vi "Read Anything.vi"(7 "Type of Anything":variant, 8 "Error In":errorcluster, 9 "Section Name (Name of \"Type of Anything\")":string, 11 "Path (dialog)":path) -> (0 "Error Out":errorcluster, 1 "Found?":bool, 3 "Anything":variant)   [LabVIEW 2009]
doc: "This VI is designed to read data from a file written by <B>Write Anything.vi</B>. If the data type definition has changed since it was written to file, this VI will still read and fill out any elements of the cluster that have the same name. Any elements for which it cannot find a name match in the file will be supplied with their datatype's default value.\n\nFreeware from Moore Good Ideas, www.mooregoodideas.com. Do not remove this line."
uses:
  <vilib>/Utility/VariantDataType/VariantType.lvlib
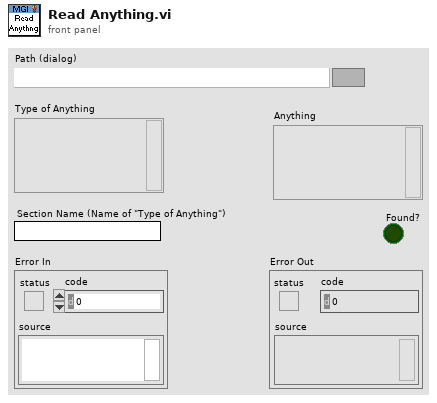
[diagram p1: front panel]
types:
  T1 = typedef "VariantType.lvlib/Type.ctl" = enum8{"Invalid Type", "Void", "I8", "I16", "I32", "I64", "U8", "U16", "U32", "U64", "Single Float", "Double Float", "Extended Float", "Single Complex", "Double Complex", "Extended Complex", "Enum U8", "Enum U16", "Enum U32", "Enum U64", "Single Float With Unit", "Double Float With Unit", "Extended Float With Unit", "Single Complex with Unit", "Double Complex with Unit", "Extended Complex with Unit", "Boolean", "String", "Path", "Picture", "Tag", "Array", "Cluster", "Variant", "LV Variant", "Waveform", "Timestamp", "Digital Waveform", "Digital Data", "ExpressData", "Refnum", "External Data", "VI", "Poly VI", "LabVIEW Class Instance", "Fixed Point"}
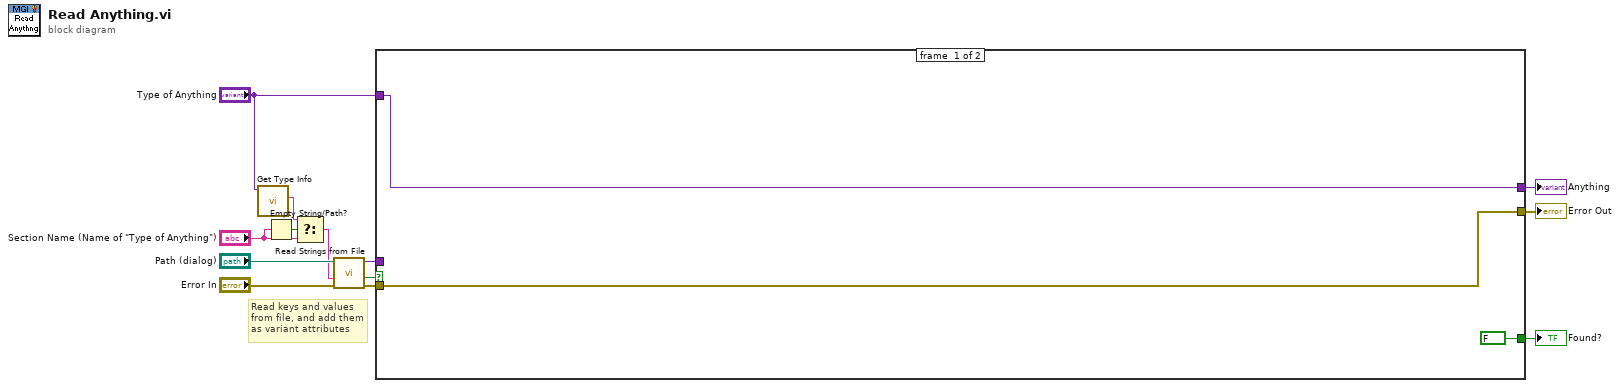
[diagram p0: block diagram]
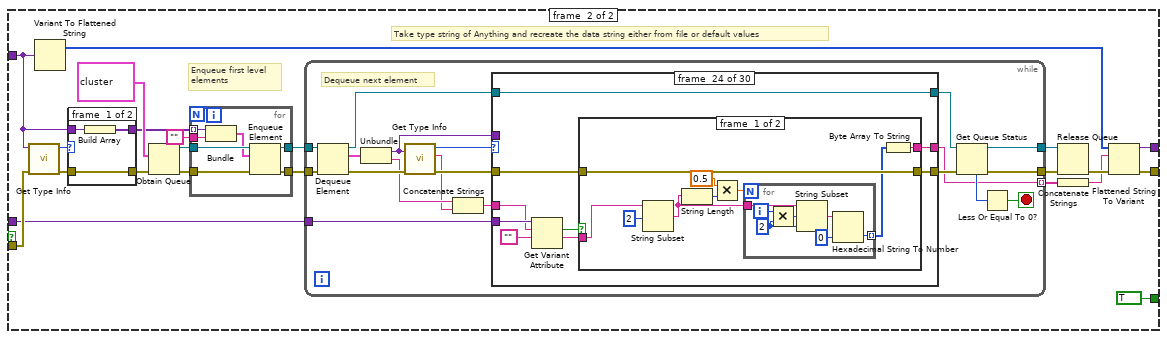
[diagram p2: hidden frame]
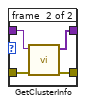
[diagram p3: hidden frame]
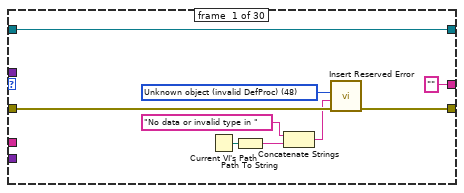
[diagram p4: hidden frame]
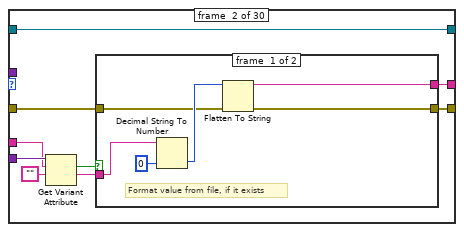
[diagram p5: hidden frame]
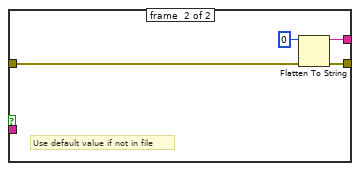
[diagram p6: hidden frame]
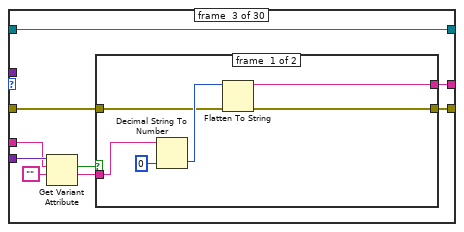
[diagram p7: hidden frame]
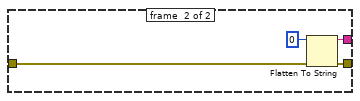
[diagram p8: hidden frame]
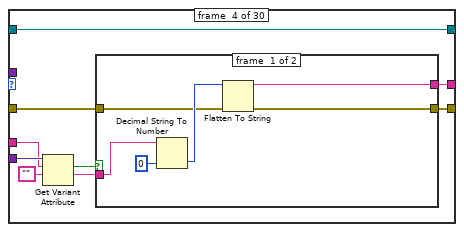
[diagram p9: hidden frame]
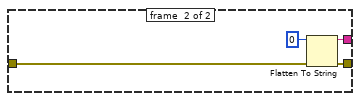
[diagram p10: hidden frame]
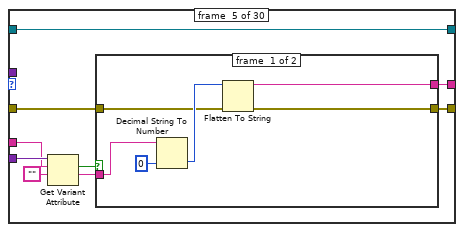
[diagram p11: hidden frame]
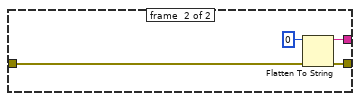
[diagram p12: hidden frame]
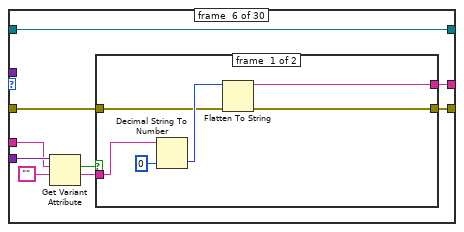
[diagram p13: hidden frame]
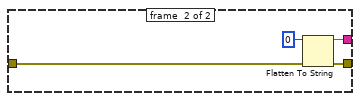
[diagram p14: hidden frame]
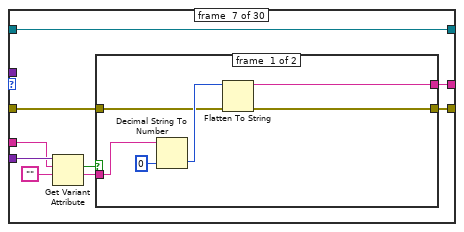
[diagram p15: hidden frame]
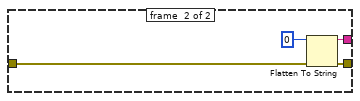
[diagram p16: hidden frame]
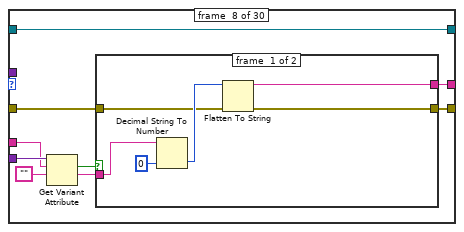
[diagram p17: hidden frame]
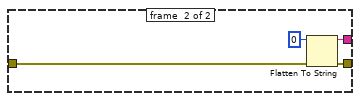
[diagram p18: hidden frame]
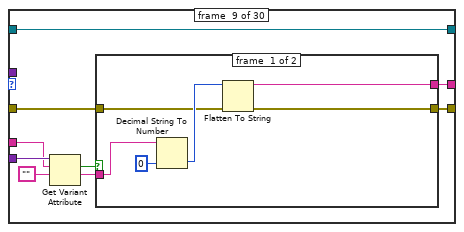
[diagram p19: hidden frame]
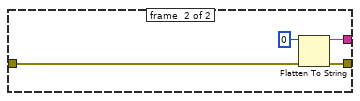
[diagram p20: hidden frame]
diagram:
  # "Read keys and values from file, and add them as variant attributes"
  n1 = call "Get Type Info.vi"("Variant"="Type of Anything") -> ("Name"=w2:string)  [unwired: 8 in, 2 out]
  n2 = Empty String/Path?(string/path="Section Name (Name of \"Type of Anything\")") -> (empty?=w5:bool)
  n3 = Select(t=w2, s=w5, f="Section Name (Name of \"Type of Anything\")") -> (s? t:f=w3:string)
  n4 = call "Read Strings from File.vi"("Error In"="Error In", "Section Name"=w3, "Path"="Path (dialog)") -> ("Error Out"=w11:errorcluster, "Found?"=w8:bool, "Variant Database"=w7:variant)  [unwired: 6 in]
  n5 = case shown="True" w8 {
    tunnel: [w15 w37] -> w13
    tunnel: [w16 w36] -> w12
    tunnel: "Type of Anything" -> [w16 w18]
    tunnel: w11 -> [w15 w24]
    tunnel: [FALSE TRUE] -> w9
    tunnel: w7 -> [_ w22]
    frame #0 {
    }
    frame #1 {
      # "Enqueue first level\nelements"
      # "Take type string of Anything and recreate the data string either from file or default values"
      n6 = call "Get Type Info.vi"("Error In"=w24, "Variant"=w18) -> ("Error Out"=w19:errorcluster, "Type Enum"=w21:T1)  [unwired: 7 in, 1 out]
      n7 = Variant To Flattened String(Variant=w18) -> (1:w38:i16[])  [unwired: 1 out]
      n8 = case shown="\"Cluster\"" w21 {
        tunnel: [w41 w44] -> w20
        tunnel: w19 -> [w41 w45]
        tunnel: w18 -> [w40 w43]
        tunnel: [w39 w42] -> w17
        frame #0 {
          n9 = Build Array(w40) -> (w39:variant[])
        }
        frame #1 {
          n10 = call <vilib>:"GetClusterInfo.vi"("error in (no error)"=w45, "Variant"=w43) -> ("error out"=w44:errorcluster, "Cluster Elements"=w42:variant[])  [unwired: 8 in]
        }
      }
      n11 = Obtain Queue(element data type=cluster{"Variant":variant, "Name":string} {"Variant"=variant, "Name"=""}, error in (no error)=w20) -> (queue out=w34:refnum<queue>, error out=w26:errorcluster)  [unwired: 3 in, 1 out]
      n12 = for {
        tunnel: w34 -> [w52]
        tunnel: [w51] -> w33
        tunnel: [w50] -> w32
        tunnel: w17 -> [w49] mode=indexing
        tunnel: "" -> [w47]
        tunnel: w26 -> [w46]
        n13 = Bundle("ArrayElt"=w49, w47) -> (w48:cluster{"ArrayElt":variant, string})  [unwired: 1 in]
        n14 = Enqueue Element(queue=w52, element=w48, error in (no error)=w46) -> (queue out=w50:refnum<queue>, error out=w51:errorcluster)  [unwired: 1 in, 1 out]
      }
      n15 = while {
        tunnel: w33 -> [w69]
        tunnel: [w64] -> w31
        tunnel: w22 -> [w56]
        tunnel: [w53] -> w35 mode=indexing
        tunnel: w32 -> [w66]
        tunnel: [w60] -> w29
        stop <- w61 stop-if-true
        # "Dequeue next element"
        n16 = Dequeue Element(queue=w66, error in (no error)=w69) -> (queue out=w67:refnum<queue>, element=w59:cluster{"Variant":variant, "Name":string}, error out=w68:errorcluster)  [unwired: 1 in, 1 out]
        n17 = Unbundle(w59) -> ("Variant"=w55:variant, "Name"=w57:string)
        n18 = call "Get Type Info.vi"("Error In"=w68, "Variant"=w55) -> ("Error Out"=w70:errorcluster, "Name"=w54:string, "Type Enum"=w71:T1)  [unwired: 7 in]
        n19 = Concatenate Strings(w57, w54) -> (w58:string)
        n20 = case shown="\"Invalid Type\", \"Void\"" w71 {
          tunnel: [w74 w89 w108 w127 w146 w165 w184 w203 w222 w241 w260 w279 w298 w317 w336 w356 w382 w408 w434 w459 w478 w495 w510 w532 w561 w590 w619 w648 w676 w688] -> w65
          tunnel: w70 -> [w75 w88 w107 w126 w145 w164 w183 w202 w221 w240 w259 w278 w297 w316 w335 w355 w381 w407 w433 w458 w477 w494 w516 w531 w560 w589 w618 w647 w677 w687]
          tunnel: w58 -> [_ w83 w102 w121 w140 w159 w177 w197 w216 w235 w253 w273 w291 w311 w331 w348 w374 w401 w427 w453 w472 w488 w506 w526 w555 w583 w611 w641 w671 w680]
          tunnel: ["" ("data string") w87 w106 w125 w144 w163 w182 w201 w220 w239 w258 w277 w296 w315 w334 w354 w380 w406 w432 w457 w476 w493 "" w530 w559 w588 w617 w646 w674 w686] -> w53
          tunnel: w55 -> [_ _ _ _ _ _ _ _ _ _ _ _ _ _ _ w353 w379 w405 w431 _ _ _ w515 _ _ _ _ _ w675 _]
          tunnel: w67 -> [w76 w86 w105 w124 w143 w162 w181 w200 w219 w238 w257 w276 w295 w314 w333 w352 w378 w404 w430 w456 w475 w492 w511 w529 w558 w587 w616 w645 w679 w685]
          tunnel: [w76 w86 w105 w124 w143 w162 w181 w200 w219 w238 w257 w276 w295 w314 w333 w352 w378 w404 w430 w456 w475 w492 w509 w529 w558 w587 w616 w645 w678 w685] -> w63
          tunnel: w56 -> [_ w84 w103 w122 w141 w160 w178 w198 w217 w237 w254 w274 w292 w312 w332 w350 w375 w402 w428 w454 w473 w489 _ w527 w556 w585 w614 w642 w672 w683]
          frame #0 {
            w72 = u16 48 items=["No error", "Argument error", "Memory is full", "Out of zone", "End of file", "File already open", "Generic file I/O error", "File not found", "File permission error", "Disk is full", "Duplicate path", "Too many files open", "System feature not enabled", "Resource file not found", "Cannot add resource", "Resource not found", "Image not found", "Image memory error", "Pen does not exist", "Config type invalid", "Config token not found", "Config parse error", "Config memory error", "Bad external code format", "Bad external code offset", "External code not present", "Null window", "Destroy window error", "Null menu", "Print aborted", "Bad print record", "Print driver error", "Windows error during printing", "Memory error during printing", "Print dialog error", "Generic print error", "Invalid device refnum", "Device not found", "Device parameter error", "Device unit error", "Cannot open device", "Device call aborted", "Generic error", "Cancelled by user", "Object ID too low", "Object ID too high", "Object not in heap", "Unknown heap", "Unknown object (invalid DefProc)", "Unknown object (DefProc not in table)", "Message out of range", "Invalid (null) method", "Unknown message", "Manager call not supported", "Bad address", "Network operation in progress", "Network operation timed out", "Connection is busy", "Network attribute not supported", "Network error", "Address in use", "System out of memory", "Connection aborted", "Connection refused", "Not connected", "Already connected", "Connection closed", "Initialization error (interapplication manager)", "Bad occurrence", "Wait on unbound occurrence handler", "Occurrence queue overflow", "Datalog type conflict", "Unused", "Unrecognized type (interapplication manager)", "Memory corrupt", "Failed to make temporary DLL", "Old CIN version", "Drag socket not found", "Failed to load drop-object", "Failed to register OLE object", "Failed to release OLE object", "Format specifier type mismatch", "Unknown format specifier", "Too few format specifiers", "Too many format specifiers", "Scan failed", "Newer CIN version", "OLE Convert", "Runtime menu error", "Password tampered", "Unknown error code"] ("Reserved Error Code")
            n21 = Current VI's Path() -> (path=w78:path)
            n22 = Path To String(path=w78) -> (string=w77:string)
            n23 = Concatenate Strings("No data or invalid type in " ("string"), w77) -> (w73:string)
            n24 = call "Insert Reserved Error.vi"("error in (no error)"=w75, "non-standard source (\"\")"=w73, "Reserved Error Code"=w72) -> ("error out"=w74:errorcluster)  [unwired: 4 in]
          }
          frame #1 {
            n25 = Get Variant Attribute(Variant=w84, name=w83, default value (empty Variant)="") -> (found=w81:bool, value=w82:string)  [unwired: 1 in, 2 out]
            n26 = case shown="True" w81 {
              tunnel: w82 -> [w90 _]
              tunnel: [w93 w96] -> w89
              tunnel: w88 -> [w92 w97]
              tunnel: [w94 w99] -> w87
              frame #0 {
                # "Format value from file, if it exists"
                n27 = Decimal String To Number(string=w90, default (0L)=i8 0 ("default (0 I32)")) -> (number=w95:i8)  [unwired: 1 in, 1 out]
                n28 = Flatten To String(anything=w95, error in (no error)=w92) -> (data string=w94:string, error out=w93:errorcluster)  [unwired: 2 in, 1 out]
              }
              frame #1 {
                # "Use default value if not in file"
                n29 = Flatten To String(anything=i8 0, error in (no error)=w97) -> (data string=w99:string, error out=w96:errorcluster)  [unwired: 2 in, 1 out]
              }
            }
          }
          frame #2 {
            n30 = Get Variant Attribute(Variant=w103, name=w102, default value (empty Variant)="") -> (found=w100:bool, value=w101:string)  [unwired: 1 in, 2 out]
            n31 = case shown="True" w100 {
              tunnel: w101 -> [w109 _]
              tunnel: [w112 w115] -> w108
              tunnel: w107 -> [w111 w116]
              tunnel: [w113 w118] -> w106
              frame #0 {
                n32 = Decimal String To Number(string=w109, default (0L)=i16 0 ("default (0 I32)")) -> (number=w114:i16)  [unwired: 1 in, 1 out]
                n33 = Flatten To String(anything=w114, error in (no error)=w111) -> (data string=w113:string, error out=w112:errorcluster)  [unwired: 2 in, 1 out]
              }
              frame #1 {
                n34 = Flatten To String(anything=i16 0, error in (no error)=w116) -> (data string=w118:string, error out=w115:errorcluster)  [unwired: 2 in, 1 out]
              }
            }
          }
          frame #3 {
            n35 = Get Variant Attribute(Variant=w122, name=w121, default value (empty Variant)="") -> (found=w119:bool, value=w120:string)  [unwired: 1 in, 2 out]
            n36 = case shown="True" w119 {
              tunnel: w120 -> [w128 _]
              tunnel: [w131 w134] -> w127
              tunnel: w126 -> [w130 w135]
              tunnel: [w132 w137] -> w125
              frame #0 {
                n37 = Decimal String To Number(string=w128, default (0L)=0 ("default (0 I32)")) -> (number=w133:i32)  [unwired: 1 in, 1 out]
                n38 = Flatten To String(anything=w133, error in (no error)=w130) -> (data string=w132:string, error out=w131:errorcluster)  [unwired: 2 in, 1 out]
              }
              frame #1 {
                n39 = Flatten To String(anything=0, error in (no error)=w135) -> (data string=w137:string, error out=w134:errorcluster)  [unwired: 2 in, 1 out]
              }
            }
          }
          frame #4 {
            n40 = Get Variant Attribute(Variant=w141, name=w140, default value (empty Variant)="") -> (found=w138:bool, value=w139:string)  [unwired: 1 in, 2 out]
            n41 = case shown="True" w138 {
              tunnel: w139 -> [w147 _]
              tunnel: [w150 w153] -> w146
              tunnel: w145 -> [w149 w154]
              tunnel: [w151 w156] -> w144
              frame #0 {
                n42 = Decimal String To Number(string=w147, default (0L)=i64 0 ("default (0 I32)")) -> (number=w152:i64)  [unwired: 1 in, 1 out]
                n43 = Flatten To String(anything=w152, error in (no error)=w149) -> (data string=w151:string, error out=w150:errorcluster)  [unwired: 2 in, 1 out]
              }
              frame #1 {
                n44 = Flatten To String(anything=i64 0, error in (no error)=w154) -> (data string=w156:string, error out=w153:errorcluster)  [unwired: 2 in, 1 out]
              }
            }
          }
          frame #5 {
            n45 = Get Variant Attribute(Variant=w160, name=w159, default value (empty Variant)="") -> (found=w157:bool, value=w158:string)  [unwired: 1 in, 2 out]
            n46 = case shown="True" w157 {
              tunnel: w158 -> [w166 _]
              tunnel: [w169 w172] -> w165
              tunnel: w164 -> [w168 w173]
              tunnel: [w170 w175] -> w163
              frame #0 {
                n47 = Decimal String To Number(string=w166, default (0L)=u8 0 ("default (0 I32)")) -> (number=w171:u8)  [unwired: 1 in, 1 out]
                n48 = Flatten To String(anything=w171, error in (no error)=w168) -> (data string=w170:string, error out=w169:errorcluster)  [unwired: 2 in, 1 out]
              }
              frame #1 {
                n49 = Flatten To String(anything=u8 0, error in (no error)=w173) -> (data string=w175:string, error out=w172:errorcluster)  [unwired: 2 in, 1 out]
              }
            }
          }
          frame #6 {
            n50 = Get Variant Attribute(Variant=w178, name=w177, default value (empty Variant)="") -> (found=w176:bool, value=w179:string)  [unwired: 1 in, 2 out]
            n51 = case shown="True" w176 {
              tunnel: w179 -> [w185 _]
              tunnel: [w188 w191] -> w184
              tunnel: w183 -> [w187 w192]
              tunnel: [w189 w194] -> w182
              frame #0 {
                n52 = Decimal String To Number(string=w185, default (0L)=u16 0 ("default (0 I32)")) -> (number=w190:u16)  [unwired: 1 in, 1 out]
                n53 = Flatten To String(anything=w190, error in (no error)=w187) -> (data string=w189:string, error out=w188:errorcluster)  [unwired: 2 in, 1 out]
              }
              frame #1 {
                n54 = Flatten To String(anything=u16 0, error in (no error)=w192) -> (data string=w194:string, error out=w191:errorcluster)  [unwired: 2 in, 1 out]
              }
            }
          }
          frame #7 {
            n55 = Get Variant Attribute(Variant=w198, name=w197, default value (empty Variant)="") -> (found=w195:bool, value=w196:string)  [unwired: 1 in, 2 out]
            n56 = case shown="True" w195 {
              tunnel: w196 -> [w204 _]
              tunnel: [w207 w210] -> w203
              tunnel: w202 -> [w206 w211]
              tunnel: [w208 w213] -> w201
              frame #0 {
                n57 = Decimal String To Number(string=w204, default (0L)=u32 0 ("default (0 I32)")) -> (number=w209:u32)  [unwired: 1 in, 1 out]
                n58 = Flatten To String(anything=w209, error in (no error)=w206) -> (data string=w208:string, error out=w207:errorcluster)  [unwired: 2 in, 1 out]
              }
              frame #1 {
                n59 = Flatten To String(anything=u32 0, error in (no error)=w211) -> (data string=w213:string, error out=w210:errorcluster)  [unwired: 2 in, 1 out]
              }
            }
          }
          frame #8 {
            n60 = Get Variant Attribute(Variant=w217, name=w216, default value (empty Variant)="") -> (found=w214:bool, value=w215:string)  [unwired: 1 in, 2 out]
            n61 = case shown="True" w214 {
              tunnel: w215 -> [w223 _]
              tunnel: [w226 w229] -> w222
              tunnel: w221 -> [w225 w230]
              tunnel: [w227 w232] -> w220
              frame #0 {
                n62 = Decimal String To Number(string=w223, default (0L)=u64 0 ("default (0 I32)")) -> (number=w228:u64)  [unwired: 1 in, 1 out]
                n63 = Flatten To String(anything=w228, error in (no error)=w225) -> (data string=w227:string, error out=w226:errorcluster)  [unwired: 2 in, 1 out]
              }
              frame #1 {
                n64 = Flatten To String(anything=u64 0, error in (no error)=w230) -> (data string=w232:string, error out=w229:errorcluster)  [unwired: 2 in, 1 out]
              }
            }
          }
          frame #9 {
            n65 = Get Variant Attribute(Variant=w237, name=w235, default value (empty Variant)="") -> (found=w233:bool, value=w234:string)  [unwired: 1 in, 2 out]
            n66 = case shown="True" w233 {
              tunnel: w234 -> [w242 _]
              tunnel: [w245 w248] -> w241
              tunnel: w240 -> [w244 w249]
              tunnel: [w246 w251] -> w239
              frame #0 {
                n67 = Fract/Exp String To Number(string=w242, default (0 dbl)=sgl 0.0 ("default (0 I32)")) -> (number=w247:sgl)  [unwired: 2 in, 1 out]
                n68 = Flatten To String(anything=w247, error in (no error)=w244) -> (data string=w246:string, error out=w245:errorcluster)  [unwired: 2 in, 1 out]
              }
              frame #1 {
                n69 = Flatten To String(anything=sgl 0.0, error in (no error)=w249) -> (data string=w251:string, error out=w248:errorcluster)  [unwired: 2 in, 1 out]
              }
            }
          }
          frame #10 {
            n70 = Get Variant Attribute(Variant=w254, name=w253, default value (empty Variant)="") -> (found=w252:bool, value=w255:string)  [unwired: 1 in, 2 out]
            n71 = case shown="True" w252 {
              tunnel: w255 -> [w261 _]
              tunnel: [w264 w267] -> w260
              tunnel: w259 -> [w263 w268]
              tunnel: [w265 w270] -> w258
              frame #0 {
                n72 = Fract/Exp String To Number(string=w261, default (0 dbl)=0.0 ("default (0 DBL)")) -> (number=w266:dbl)  [unwired: 2 in, 1 out]
                n73 = Flatten To String(anything=w266, error in (no error)=w263) -> (data string=w265:string, error out=w264:errorcluster)  [unwired: 2 in, 1 out]
              }
              frame #1 {
                n74 = Flatten To String(anything=0.0, error in (no error)=w268) -> (data string=w270:string, error out=w267:errorcluster)  [unwired: 2 in, 1 out]
              }
            }
          }
          frame #11 {
            n75 = Get Variant Attribute(Variant=w274, name=w273, default value (empty Variant)="") -> (found=w271:bool, value=w272:string)  [unwired: 1 in, 2 out]
            n76 = case shown="True" w271 {
              tunnel: w272 -> [w280 _]
              tunnel: [w283 w286] -> w279
              tunnel: w278 -> [w282 w287]
              tunnel: [w284 w289] -> w277
              frame #0 {
                n77 = Fract/Exp String To Number(string=w280, default (0 dbl)=ext 0.0 ("default (0 DBL)")) -> (number=w285:ext)  [unwired: 2 in, 1 out]
                n78 = Flatten To String(anything=w285, error in (no error)=w282) -> (data string=w284:string, error out=w283:errorcluster)  [unwired: 2 in, 1 out]
              }
              frame #1 {
                n79 = Flatten To String(anything=ext 0.0, error in (no error)=w287) -> (data string=w289:string, error out=w286:errorcluster)  [unwired: 2 in, 1 out]
              }
            }
          }
          frame #12 {
            n80 = Get Variant Attribute(Variant=w292, name=w291, default value (empty Variant)="") -> (found=w290:bool, value=w293:string)  [unwired: 1 in, 2 out]
            n81 = case shown="True" w290 {
              tunnel: w293 -> [w299 _]
              tunnel: [w303 w305] -> w298
              tunnel: w297 -> [w302 w306]
              tunnel: [w304 w308] -> w296
              frame #0 {
                n82 = Scan From String(input string=w299, default 1=csg 0.0+0.0i ("default (0 DBL)")) -> (output 1=w300:csg)  [unwired: 3 in, 3 out]
                n83 = Flatten To String(anything=w300, error in (no error)=w302) -> (data string=w304:string, error out=w303:errorcluster)  [unwired: 2 in, 1 out]
              }
              frame #1 {
                n84 = Flatten To String(anything=csg 0.0+0.0i, error in (no error)=w306) -> (data string=w308:string, error out=w305:errorcluster)  [unwired: 2 in, 1 out]
              }
            }
          }
          frame #13 {
            n85 = Get Variant Attribute(Variant=w312, name=w311, default value (empty Variant)="") -> (found=w309:bool, value=w310:string)  [unwired: 1 in, 2 out]
            n86 = case shown="True" w309 {
              tunnel: w310 -> [w318 _]
              tunnel: [w322 w324] -> w317
              tunnel: w316 -> [w321 w325]
              tunnel: [w323 w327] -> w315
              frame #0 {
                n87 = Scan From String(input string=w318, default 1=cdb 0.0+0.0i ("default (0 DBL)")) -> (output 1=w320:cdb)  [unwired: 3 in, 3 out]
                n88 = Flatten To String(anything=w320, error in (no error)=w321) -> (data string=w323:string, error out=w322:errorcluster)  [unwired: 2 in, 1 out]
              }
              frame #1 {
                n89 = Flatten To String(anything=cdb 0.0+0.0i, error in (no error)=w325) -> (data string=w327:string, error out=w324:errorcluster)  [unwired: 2 in, 1 out]
              }
            }
          }
          frame #14 {
            n90 = Get Variant Attribute(Variant=w332, name=w331, default value (empty Variant)="") -> (found=w328:bool, value=w329:string)  [unwired: 1 in, 2 out]
            n91 = case shown="True" w328 {
              tunnel: w329 -> [w337 _]
              tunnel: [w341 w343] -> w336
              tunnel: w335 -> [w340 w344]
              tunnel: [w342 w346] -> w334
              frame #0 {
                n92 = Scan From String(input string=w337, default 1=cxt 0.0+0.0i ("default (0 DBL)")) -> (output 1=w338:cxt)  [unwired: 3 in, 3 out]
                n93 = Flatten To String(anything=w338, error in (no error)=w340) -> (data string=w342:string, error out=w341:errorcluster)  [unwired: 2 in, 1 out]
              }
              frame #1 {
                n94 = Flatten To String(anything=cxt 0.0+0.0i, error in (no error)=w344) -> (data string=w346:string, error out=w343:errorcluster)  [unwired: 2 in, 1 out]
              }
            }
          }
          frame #15 {
            n95 = Get Variant Attribute(Variant=w350, name=w348, default value (empty Variant)="") -> (found=w347:bool, value=w349:string)  [unwired: 1 in, 2 out]
            n96 = case shown="True" w347 {
              tunnel: w349 -> [w357 _]
              tunnel: [w367 w370] -> w356
              tunnel: w355 -> [w366 w371]
              tunnel: [w368 w372] -> w354
              tunnel: w353 -> [w365 _]
              frame #0 {
                n97 = call <vilib>:"GetNumericInfo.vi"("error in (no error)"=w366, "Variant"=w365) -> ("error out"=w358:errorcluster, "EnumNames"=w364:string[])  [unwired: 7 in, 1 out]
                n98 = Search 1D Array(1D array=w364, element=w357) -> (index of element=w363:i32)  [unwired: 1 in]
                n99 = In Range and Coerce(upper limit=255, x=w363, lower limit=0) -> (coerced(x)=w361:i32)  [unwired: 1 out]
                n100 = To Unsigned Byte Integer(number=w361) -> (unsigned 8bit integer=w362:u8)
                n101 = Flatten To String(anything=w362, error in (no error)=w358) -> (data string=w368:string, error out=w367:errorcluster)  [unwired: 2 in, 1 out]
              }
              frame #1 {
                n102 = Flatten To String(anything=u8 0, error in (no error)=w371) -> (data string=w372:string, error out=w370:errorcluster)  [unwired: 2 in, 1 out]
              }
            }
          }
          frame #16 {
            n103 = Get Variant Attribute(Variant=w375, name=w374, default value (empty Variant)="") -> (found=w373:bool, value=w376:string)  [unwired: 1 in, 2 out]
            n104 = case shown="True" w373 {
              tunnel: w376 -> [w383 _]
              tunnel: [w393 w396] -> w382
              tunnel: w381 -> [w392 w397]
              tunnel: [w394 w398] -> w380
              tunnel: w379 -> [w391 _]
              frame #0 {
                n105 = call <vilib>:"GetNumericInfo.vi"("error in (no error)"=w392, "Variant"=w391) -> ("error out"=w384:errorcluster, "EnumNames"=w390:string[])  [unwired: 7 in, 1 out]
                n106 = Search 1D Array(1D array=w390, element=w383) -> (index of element=w389:i32)  [unwired: 1 in]
                n107 = In Range and Coerce(upper limit=u16 65535, x=w389, lower limit=0) -> (coerced(x)=w387:i32)  [unwired: 1 out]
                n108 = To Unsigned Word Integer(number=w387) -> (unsigned 16bit integer=w388:u16)
                n109 = Flatten To String(anything=w388, error in (no error)=w384) -> (data string=w394:string, error out=w393:errorcluster)  [unwired: 2 in, 1 out]
              }
              frame #1 {
                n110 = Flatten To String(anything=u16 0, error in (no error)=w397) -> (data string=w398:string, error out=w396:errorcluster)  [unwired: 2 in, 1 out]
              }
            }
          }
          frame #17 {
            n111 = Get Variant Attribute(Variant=w402, name=w401, default value (empty Variant)="") -> (found=w399:bool, value=w400:string)  [unwired: 1 in, 2 out]
            n112 = case shown="True" w399 {
              tunnel: w400 -> [w409 _]
              tunnel: [w419 w422] -> w408
              tunnel: w407 -> [w418 w423]
              tunnel: [w420 w424] -> w406
              tunnel: w405 -> [w417 _]
              frame #0 {
                n113 = call <vilib>:"GetNumericInfo.vi"("error in (no error)"=w418, "Variant"=w417) -> ("error out"=w410:errorcluster, "EnumNames"=w416:string[])  [unwired: 7 in, 1 out]
                n114 = Search 1D Array(1D array=w416, element=w409) -> (index of element=w415:i32)  [unwired: 1 in]
                n115 = In Range and Coerce(upper limit=u32 4294967295, x=w415, lower limit=0) -> (coerced(x)=w413:u32)  [unwired: 1 out]
                n116 = To Unsigned Long Integer(number=w413) -> (unsigned 32bit integer=w414:u32)
                n117 = Flatten To String(anything=w414, error in (no error)=w410) -> (data string=w420:string, error out=w419:errorcluster)  [unwired: 2 in, 1 out]
              }
              frame #1 {
                n118 = Flatten To String(anything=u32 0, error in (no error)=w423) -> (data string=w424:string, error out=w422:errorcluster)  [unwired: 2 in, 1 out]
              }
            }
          }
          frame #18 {
            n119 = Get Variant Attribute(Variant=w428, name=w427, default value (empty Variant)="") -> (found=w425:bool, value=w426:string)  [unwired: 1 in, 2 out]
            n120 = case shown="True" w425 {
              tunnel: [w445 w448] -> w434
              tunnel: w433 -> [w444 w449]
              tunnel: [w446 w450] -> w432
              tunnel: w431 -> [w443 _]
              tunnel: w426 -> [w435 _]
              frame #0 {
                n121 = call <vilib>:"GetNumericInfo.vi"("error in (no error)"=w444, "Variant"=w443) -> ("error out"=w436:errorcluster, "EnumNames"=w442:string[])  [unwired: 7 in, 1 out]
                n122 = Search 1D Array(1D array=w442, element=w435) -> (index of element=w441:i32)  [unwired: 1 in]
                n123 = In Range and Coerce(upper limit=u64 18446744073709551615, x=w441, lower limit=0) -> (coerced(x)=w439:u64)  [unwired: 1 out]
                n124 = To Unsigned Quad Integer(1:w439) -> (0:w440:u64)
                n125 = Flatten To String(anything=w440, error in (no error)=w436) -> (data string=w446:string, error out=w445:errorcluster)  [unwired: 2 in, 1 out]
              }
              frame #1 {
                n126 = Flatten To String(anything=u64 0, error in (no error)=w449) -> (data string=w450:string, error out=w448:errorcluster)  [unwired: 2 in, 1 out]
              }
            }
          }
          frame #19 {
            n127 = Get Variant Attribute(Variant=w454, name=w453, default value (empty Variant)="") -> (found=w451:bool, value=w452:string)  [unwired: 1 in, 2 out]
            n128 = case shown="True" w451 {
              tunnel: w452 -> [w460 _]
              tunnel: [w464 w467] -> w459
              tunnel: w458 -> [w461 w468]
              tunnel: [w465 w469] -> w457
              frame #0 {
                n129 = Equal?(x=w460, y="TRUE") -> (x = y?=w462:bool)
                n130 = Flatten To String(anything=w462, error in (no error)=w461) -> (data string=w465:string, error out=w464:errorcluster)  [unwired: 2 in, 1 out]
              }
              frame #1 {
                n131 = Flatten To String(anything=FALSE, error in (no error)=w468) -> (data string=w469:string, error out=w467:errorcluster)  [unwired: 2 in, 1 out]
              }
            }
          }
          frame #20 {
            n132 = Get Variant Attribute(Variant=w473, name=w472, default value (empty Variant)="") -> (found=w471:bool, value=w470:string)  [unwired: 1 in, 2 out]
            n133 = case shown="True" w471 {
              tunnel: [w481 w484] -> w478
              tunnel: w477 -> [w480 w485]
              tunnel: [w482 w486] -> w476
              tunnel: w470 -> [w479 _]
              frame #0 {
                n134 = Flatten To String(anything=w479, error in (no error)=w480) -> (data string=w482:string, error out=w481:errorcluster)  [unwired: 2 in, 1 out]
              }
              frame #1 {
                n135 = Flatten To String(anything="", error in (no error)=w485) -> (data string=w486:string, error out=w484:errorcluster)  [unwired: 2 in, 1 out]
              }
            }
          }
          frame #21 {
            n136 = Get Variant Attribute(Variant=w489, name=w488, default value (empty Variant)="") -> (found=w490:bool, value=w487:string)  [unwired: 1 in, 2 out]
            n137 = case shown="True" w490 {
              tunnel: [w499 w502] -> w495
              tunnel: w494 -> [w498 w503]
              tunnel: [w500 w504] -> w493
              tunnel: w487 -> [w496 _]
              frame #0 {
                n138 = String To Path(string=w496) -> (path=w497:path)
                n139 = Flatten To String(anything=w497, error in (no error)=w498) -> (data string=w500:string, error out=w499:errorcluster)  [unwired: 2 in, 1 out]
              }
              frame #1 {
                n140 = Flatten To String(anything=path "", error in (no error)=w503) -> (data string=w504:string, error out=w502:errorcluster)  [unwired: 2 in, 1 out]
              }
            }
          }
          frame #22 {
            # "Enqueue cluster elements"
            n141 = call <vilib>:"GetClusterInfo.vi"("error in (no error)"=w516, "Variant"=w515) -> ("error out"=w512:errorcluster, "Cluster Elements"=w514:variant[])  [unwired: 8 in]
            n142 = Concatenate Strings(w506, "." ("string")) -> (w505:string)
            n143 = Reverse 1D Array(array=w514) -> (reversed array=w513:variant[])
            n144 = for {
              tunnel: w511 -> [w523]
              tunnel: w512 -> [w522]
              tunnel: [w521] -> w510
              tunnel: [w520] -> w509
              tunnel: w513 -> [w519] mode=indexing
              tunnel: w505 -> [w517]
              n145 = Bundle("ArrayElt"=w519, w517) -> (w518:cluster{"ArrayElt":variant, string})  [unwired: 1 in]
              n146 = Enqueue Element At Opposite End(queue=w523, element=w518, error in (no error)=w522) -> (queue out=w520:refnum<queue>, error out=w521:errorcluster)  [unwired: 1 in, 1 out]
            }
          }
          frame #23 {
            n147 = Get Variant Attribute(Variant=w527, name=w526, default value (empty Variant)="") -> (found=w524:bool, value=w525:string)  [unwired: 1 in, 2 out]
            n148 = case shown="True" w524 {
              tunnel: w525 -> [w533 _]
              tunnel: [w541 w550] -> w532
              tunnel: w531 -> [w541 w551]
              tunnel: [w539 w552] -> w530
              frame #0 {
                n149 = String Subset(string=w533, offset (0)=2) -> (substring=w538:string)  [unwired: 1 in]
                n150 = String Length(string=w538) -> (length=w536:i32)
                n151 = Multiply(x=0.5, y=w536) -> (x*y=w535:dbl)
                n152 = for {
                  N: w535 -> [_]
                  tunnel: w538 -> [w545]
                  tunnel: [w547] -> w537 mode=indexing
                  i -> [w544]
                  w543 = 2 ("length (rest)")
                  n153 = Multiply(x=w544, y=w543) -> (x*y=w542:i32)
                  n154 = String Subset(string=w545, offset (0)=w542, length (rest)=w543) -> (substring=w546:string)
                  n155 = Hexadecimal String To Number(string=w546, default (0uL)=u8 0 ("default (0 U32)")) -> (number=w547:u8)  [unwired: 1 in, 1 out]
                }
                n156 = Byte Array To String(unsigned byte array=w537) -> (string=w539:string)
              }
              frame #1 {
                w549 = variant  # Variant
                n157 = Flatten To String(anything=w549, error in (no error)=w551) -> (data string=w552:string, error out=w550:errorcluster)  [unwired: 2 in, 1 out]
              }
            }
          }
          frame #24 {
            n158 = Get Variant Attribute(Variant=w556, name=w555, default value (empty Variant)="") -> (found=w553:bool, value=w554:string)  [unwired: 1 in, 2 out]
            n159 = case shown="False" w553 {
              tunnel: w554 -> [w562 _]
              tunnel: [w570 w580] -> w561
              tunnel: w560 -> [w570 w579]
              tunnel: [w568 w581] -> w559
              frame #0 {
                n160 = String Subset(string=w562, offset (0)=2) -> (substring=w567:string)  [unwired: 1 in]
                n161 = String Length(string=w567) -> (length=w565:i32)
                n162 = Multiply(x=0.5, y=w565) -> (x*y=w564:dbl)
                n163 = for {
                  N: w564 -> [_]
                  tunnel: w567 -> [w574]
                  tunnel: [w576] -> w566 mode=indexing
                  i -> [w573]
                  w572 = 2 ("length (rest)")
                  n164 = Multiply(x=w573, y=w572) -> (x*y=w571:i32)
                  n165 = String Subset(string=w574, offset (0)=w571, length (rest)=w572) -> (substring=w575:string)
                  n166 = Hexadecimal String To Number(string=w575, default (0uL)=u8 0 ("default (0 U32)")) -> (number=w576:u8)  [unwired: 1 in, 1 out]
                }
                n167 = Byte Array To String(unsigned byte array=w566) -> (string=w568:string)
              }
              frame #1 {
                n168 = Flatten To String(anything=waveform(dbl) {"t0"=timestamp(0 s since 1904-01-01), "dt"=0.0, "Y"=[]} ("Waveform 2"), error in (no error)=w579) -> (data string=w581:string, error out=w580:errorcluster)  [unwired: 2 in, 1 out]
              }
            }
          }
          frame #25 {
            n169 = Get Variant Attribute(Variant=w585, name=w583, default value (empty Variant)="") -> (found=w582:bool, value=w584:string)  [unwired: 1 in, 2 out]
            n170 = case shown="False" w582 {
              tunnel: w584 -> [w591 _]
              tunnel: [w599 w609] -> w590
              tunnel: w589 -> [w599 w608]
              tunnel: [w597 w610] -> w588
              frame #0 {
                n171 = String Subset(string=w591, offset (0)=2) -> (substring=w596:string)  [unwired: 1 in]
                n172 = String Length(string=w596) -> (length=w594:i32)
                n173 = Multiply(x=0.5, y=w594) -> (x*y=w593:dbl)
                n174 = for {
                  N: w593 -> [_]
                  tunnel: w596 -> [w603]
                  tunnel: [w605] -> w595 mode=indexing
                  i -> [w602]
                  w601 = 2 ("length (rest)")
                  n175 = Multiply(x=w602, y=w601) -> (x*y=w600:i32)
                  n176 = String Subset(string=w603, offset (0)=w600, length (rest)=w601) -> (substring=w604:string)
                  n177 = Hexadecimal String To Number(string=w604, default (0uL)=u8 0 ("default (0 U32)")) -> (number=w605:u8)  [unwired: 1 in, 1 out]
                }
                n178 = Byte Array To String(unsigned byte array=w595) -> (string=w597:string)
              }
              frame #1 {
                n179 = Flatten To String(anything=timestamp(0 s since 1904-01-01), error in (no error)=w608) -> (data string=w610:string, error out=w609:errorcluster)  [unwired: 2 in, 1 out]
              }
            }
          }
          frame #26 {
            n180 = Get Variant Attribute(Variant=w614, name=w611, default value (empty Variant)="") -> (found=w612:bool, value=w613:string)  [unwired: 1 in, 2 out]
            n181 = case shown="False" w612 {
              tunnel: w613 -> [w620 _]
              tunnel: [w628 w638] -> w619
              tunnel: w618 -> [w628 w637]
              tunnel: [w626 w639] -> w617
              frame #0 {
                n182 = String Subset(string=w620, offset (0)=2) -> (substring=w625:string)  [unwired: 1 in]
                n183 = String Length(string=w625) -> (length=w623:i32)
                n184 = Multiply(x=0.5, y=w623) -> (x*y=w622:dbl)
                n185 = for {
                  N: w622 -> [_]
                  tunnel: w625 -> [w632]
                  tunnel: [w634] -> w624 mode=indexing
                  i -> [w631]
                  w630 = 2 ("length (rest)")
                  n186 = Multiply(x=w631, y=w630) -> (x*y=w629:i32)
                  n187 = String Subset(string=w632, offset (0)=w629, length (rest)=w630) -> (substring=w633:string)
                  n188 = Hexadecimal String To Number(string=w633, default (0uL)=u8 0 ("default (0 U32)")) -> (number=w634:u8)  [unwired: 1 in, 1 out]
                }
                n189 = Byte Array To String(unsigned byte array=w624) -> (string=w626:string)
              }
              frame #1 {
                n190 = call <vilib>:"DWDT Empty Digital.vi"() -> ("digital waveform out"=w636:digitalwaveform)  [unwired: 5 in]
                n191 = Flatten To String(anything=w636, error in (no error)=w637) -> (data string=w639:string, error out=w638:errorcluster)  [unwired: 2 in, 1 out]
              }
            }
          }
          frame #27 {
            n192 = Get Variant Attribute(Variant=w642, name=w641, default value (empty Variant)="") -> (found=w640:bool, value=w643:string)  [unwired: 1 in, 2 out]
            n193 = case shown="True" w640 {
              tunnel: w643 -> [w649 _]
              tunnel: [w657 w667] -> w648
              tunnel: w647 -> [w657 w666]
              tunnel: [w655 w668] -> w646
              frame #0 {
                n194 = String Subset(string=w649, offset (0)=2) -> (substring=w654:string)  [unwired: 1 in]
                n195 = String Length(string=w654) -> (length=w652:i32)
                n196 = Multiply(x=0.5, y=w652) -> (x*y=w651:dbl)
                n197 = for {
                  N: w651 -> [_]
                  tunnel: w654 -> [w661]
                  tunnel: [w663] -> w653 mode=indexing
                  i -> [w660]
                  w659 = 2 ("length (rest)")
                  n198 = Multiply(x=w660, y=w659) -> (x*y=w658:i32)
                  n199 = String Subset(string=w661, offset (0)=w658, length (rest)=w659) -> (substring=w662:string)
                  n200 = Hexadecimal String To Number(string=w662, default (0uL)=u8 0 ("default (0 U32)")) -> (number=w663:u8)  [unwired: 1 in, 1 out]
                }
                n201 = Byte Array To String(unsigned byte array=w653) -> (string=w655:string)
              }
              frame #1 {
                n202 = call <vilib>:"DTbl Empty Digital.vi"() -> ("digital data"=w665:digitaldata)  [unwired: 5 in]
                n203 = Flatten To String(anything=w665, error in (no error)=w666) -> (data string=w668:string, error out=w667:errorcluster)  [unwired: 2 in, 1 out]
              }
            }
          }
          frame #28 {
            n204 = Get Variant Attribute(Variant=w672, name=w671, default value (empty Variant)="") -> (duplicate Variant=w669:variant, value=w670:string)  [unwired: 1 in, 2 out]
            n205 = call "Unprocess Array Elements.vi"("Variant Database"=w669, "Value"=w670, "Error In"=w677, "Name In"=w671, "Array Variant"=w675, "Queue In"=w679) -> ("Error Out"=w676:errorcluster, "Data Out"=w674:string, "Queue Out"=w678:refnum<queue>)  [unwired: 3 in]
          }
          frame #29 {
            n206 = Get Variant Attribute(Variant=w683, name=w680, default value (empty Variant)="") -> (found=w681:bool, value=w682:string)  [unwired: 1 in, 2 out]
            n207 = case shown="True" w681 {
              tunnel: w682 -> [w689 _]
              tunnel: [w697 w706] -> w688
              tunnel: w687 -> [w697 w707]
              tunnel: [w695 w708] -> w686
              frame #0 {
                n208 = String Subset(string=w689, offset (0)=2) -> (substring=w694:string)  [unwired: 1 in]
                n209 = String Length(string=w694) -> (length=w692:i32)
                n210 = Multiply(x=0.5, y=w692) -> (x*y=w690:dbl)
                n211 = for {
                  N: w690 -> [_]
                  tunnel: w694 -> [w701]
                  tunnel: [w703] -> w693 mode=indexing
                  i -> [w700]
                  w699 = 2 ("length (rest)")
                  n212 = Multiply(x=w700, y=w699) -> (x*y=w698:i32)
                  n213 = String Subset(string=w701, offset (0)=w698, length (rest)=w699) -> (substring=w702:string)
                  n214 = Hexadecimal String To Number(string=w702, default (0uL)=u8 0 ("default (0 U32)")) -> (number=w703:u8)  [unwired: 1 in, 1 out]
                }
                n215 = Byte Array To String(unsigned byte array=w693) -> (string=w695:string)
              }
              frame #1 {
                n216 = Flatten To String(anything="", error in (no error)=w707) -> (data string=w708:string, error out=w706:errorcluster)  [unwired: 2 in, 1 out]
              }
            }
          }
        }
        n217 = Get Queue Status(queue=w63, error in (no error)=w65) -> (queue out=w60:refnum<queue>, error out=w64:errorcluster, # elements in queue=w62:i32)  [unwired: 1 in, 5 out]
        n218 = Less Or Equal To 0?(x=w62) -> (x <= 0?=w61:bool)
      }
      n219 = Release Queue(queue=w29, error in (no error)=w31) -> (error out=w30:errorcluster)  [unwired: 1 in, 2 out]
      n220 = Concatenate Strings(w35) -> (w23:string)
      n221 = Flattened String To Variant(4:w30, 6:w23, 7:w38) -> (0:w37:errorcluster, 3:w36:variant)
    }
  }
  "Error Out" <- w13
  "Anything" <- w12
  "Found?" <- w9
